vi "矩阵数据.vi"(10 "数值":i32, 11 "数据":dbl[](array[numeric])) -> (2 "强度矩阵":dbl[][](array[numeric]), 3 "原始矩阵":dbl[][](array[numeric]))   [LabVIEW 2011]
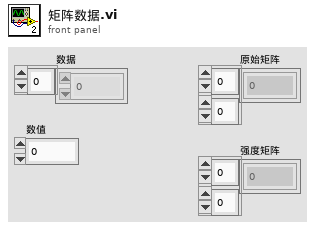
[diagram p1: front panel]
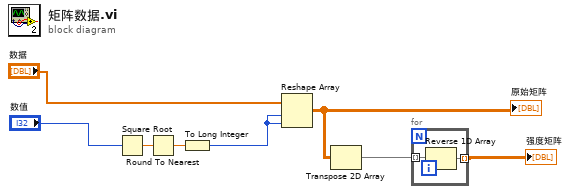
[diagram p0: block diagram]
diagram:
  n1 = Square Root(x="数值") -> (sqrt(x)=w4:dbl)
  n2 = Round To Nearest(number=w4) -> (nearest integer value=w3:dbl)
  n3 = To Long Integer(number=w3) -> (32bit integer=w1:i32)
  n4 = Reshape Array("数据", w1, w1) -> (w5:dbl[][])
  "原始矩阵" <- w5
  n5 = Transpose 2D Array(2D array=w5) -> (transposed array=w6:dbl[][])
  n6 = for {
    tunnel: w6 -> [w10] mode=indexing
    tunnel: [w9] -> w7 mode=indexing
    n7 = Reverse 1D Array(array=w10) -> (reversed array=w9:dbl[])
  }
  "强度矩阵" <- w7
